vi "Histogram.vi"(10 "intervals":i32=10, 11 "X":dbl[](array[numeric]) format="%0.2f") -> (0 "error":i32, 1 "X Values":dbl[](array[numeric]) format="%0.2f", 2 "Histogram: h(x)":i32[](array[numeric]), 3 "Histogram Graph":T1(graph))   [LabVIEW 2020, in "NI_AALBase.lvlib"]
doc: "Finds the discrete histogram of the input sequence <B>X</B>."
uses:
  NI_AALBase.lvlib
  <resource>/lvanlys.dll
panel:
  # "Histogram"
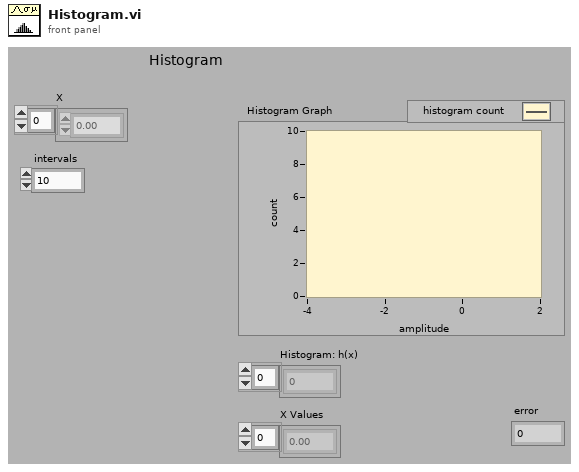
[diagram p1: front panel]
types:
  T1 = cluster{"X Values":dbl[], "Histogram: h(x)":i32[]}
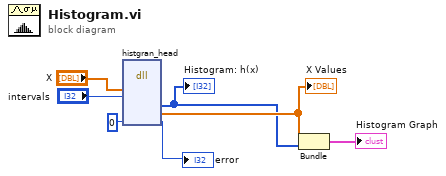
[diagram p0: block diagram]
diagram:
  n1 = dll-call lib="C:/Program Files (x86)/National Instruments/LabVIEW 2020/resource/lvanlys.*" fn="histgran_head"("X"="X", "intervals"="intervals", "error"=0) -> ("Histogram: h(x)"=w2:i32[], "X Values"=w3:dbl[], "error"=→"error":i32)  [unwired: 8 in, 2 out]
  "Histogram: h(x)" <- w2
  "X Values" <- w3
  n2 = Bundle("X Values"=w3, "Histogram: h(x)"=w2) -> (→"Histogram Graph":T1)  [unwired: 1 in]
